vi "Celsius Temperature Simulator.vi"(11 "error in (no error)":errorcluster) -> (4 "Temperature":dbl, 15 "error out":errorcluster)   [LabVIEW 2010]
doc: "Generates a simulated random temperature between 20 and 30 degrees Celsius."
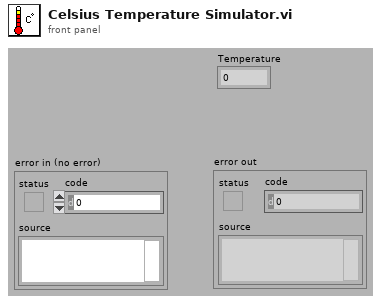
[diagram p1: front panel]
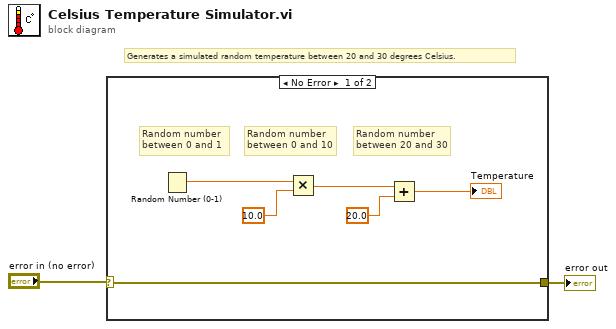
[diagram p0: block diagram]
diagram:
  # "Generates a simulated random temperature between 20 and 30 degrees Celsius."
  n1 = case shown="No Error" "error in (no error)" {
    selector: "error in (no error)" -> [w3 w9]
    tunnel: [w3 w9] -> w1
    frame No Error {
      # "Random number between 20 and 30"
      # "Random number between 0 and 10"
      # "Random number between 0 and 1"
      n2 = Random Number (0-1)() -> (number: 0 to 1=w8:dbl)
      n3 = Multiply(x=w8, y=10.0) -> (x*y=w6:dbl)
      n4 = Add(x=w6, y=20.0) -> (x+y=→"Temperature":dbl)
    }
    frame Error {
    }
  }
  "error out" <- w1
